vi "Teardown.vi"(11 "Event Actor in":refnum<class "Event Actor.lvclass">) -> (0 "error out":errorcluster)   [LabVIEW 2021, in "Event Actor.lvclass"]
uses:
  Event Actor.lvclass
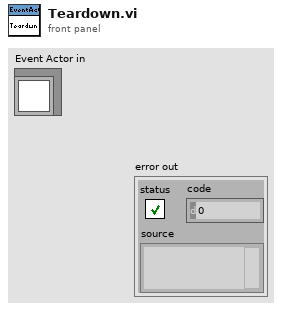
[diagram p1: front panel]
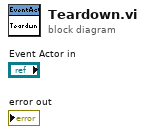
[diagram p0: block diagram]
diagram:
